vi "Return Button State Method.vi"(0 "Display State In":T2={"Buttons Displayed"=0, "Button States"=[], "Button Size"=0, "Button Style"=enum."Classic", "Active Button"=0, "Force Regen?"=FALSE, "Tip String Ref"=refnum}, 5 "Index":variant, 9 "Container State":T4, 11 "error in (no error)":errorcluster) -> (4 "Display State Out":T2={"Buttons Displayed"=0, "Button States"=[], "Button Size"=0, "Button Style"=enum."Classic", "Active Button"=0, "Force Regen?"=FALSE, "Tip String Ref"=refnum}, 6 "State":T1, 15 "error out":errorcluster)   [LabVIEW 2012, in "Toolbar.xctl"]
doc: "Returns the state of a particiular button, indexed wither by name or number"
uses:
  Toolbar.xctl
  <vilib>/_xctls/Container State.ctl
  Toolbar State.ctl
  Button_Class/Button.lvclass
  Button_Class/Type Defs/Button Style.ctl
  Button_Class/Type Defs/Button Status.ctl
  <vilib>/_xctls/XControlSupport.lvlib
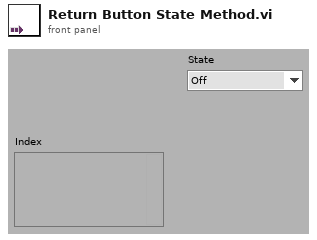
[diagram p1: front panel]
types:
  T1 = typedef "Button.lvclass/Button Status.ctl" = enum16{"Off", "Hover", "On", "Disabled"}
  T2 = typedef "Toolbar.xctl/Toolbar State.ctl" = cluster{"Buttons Displayed":i32, "Button States":refnum<class "Button.lvclass">[], "Button Size":i32, "Button Style":T3, "Active Button":i32, "Force Regen?":bool, "Tip String Ref":refnum<vi>}
  T3 = typedef "Button.lvclass/Button Style.ctl" = enum16{"System", "Modern", "Classic", "Rounded", "Silver", "Ni Theme", "Metallic"}
  T4 = typedef "XControlSupport.lvlib/Container State.ctl" = cluster{"Indicator?":bool, "Run Mode?":bool, " Refnum":refnum<vi>}
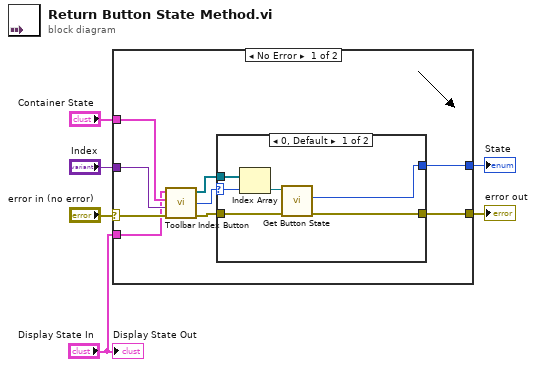
[diagram p0: block diagram]
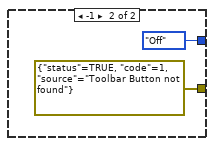
[diagram p2: hidden frame]
diagram:
  n1 = case shown="No Error" "error in (no error)" {
    selector: "error in (no error)" -> [w14 w24]
    tunnel: "Index" -> [w15 _]
    tunnel: [w10 _] -> w4
    tunnel: [w9 w24] -> w3
    tunnel: "Display State In" -> [w7 _]
    tunnel: "Container State" -> [w8 _]
    frame No Error {
      n2 = call "Toolbar Index Button.vi"("error In (no error)"=w14, "Index"=w15, "Container State"=w8, 10:w7) -> ("error out"=w11:errorcluster, "Output"=w13:refnum<class "Button.lvclass">[], "index of element"=w12:i32)  [unwired: 4 in]
      n3 = case shown="0, Default" w12 {
        selector: w12 -> [w20 _]
        tunnel: w13 -> [w21 _]
        tunnel: w11 -> [w18 _]
        tunnel: [w17 Button_Status."Off" ("State")] -> w10
        tunnel: [w16 errorcluster {"status"=TRUE, "code"=1, "source"="Toolbar Button not found"} ("error out")] -> w9
        frame 0, Default {
          n4 = Index Array(array=w21, index=w20) -> (element=w19:refnum<class "Button.lvclass">)
          n5 = call-dynamic "Get Button State.vi"("error in (no error)"=w18, "Button in"=w19) -> ("error out"=w16:errorcluster, "State"=w17:T1)  [unwired: 8 out]
        }
        frame -1 {
        }
      }
    }
    frame Error {
    }
  }
  "error out" <- w3
  "State" <- w4
  "Display State Out" <- "Display State In"
